vi "Open FTDI.vi"(8 "Baud Rate":u32=50000) -> (0 "FT_Status":u32(ring) items=["FT_OK", "FT_INVALID_HANDLE", "FT_DEVICE_NOT_FOUND", "FT_DEVICE_NOT_OPENED", "FT_IO_ERROR", "FT_INSUFFICIENT_RESOURCES", "FT_INVALID_PARAMETER", "FT_INVALID_BAUD_RATE", "FT_DEVICE_NOT_OPENED_FOR_ERASE", "FT_DEVICE_NOT_OPENED_FOR_WRITE", "FT_FAILED_TO_WRITE_DEVICE", "FT_EEPROM_READ_FAILED", "FT_EEPROM_WRITE_FAILED", "FT_EEPROM_ERASE_FAILED", "FT_EEPROM_NOT_PRESENT", "FT_EEPROM_NOT_PROGRAMMED", "FT_INVALID_ARGS", "FT_NOT_SUPPORTED", "FT_OTHER_ERROR"], 3 "FTDI Handle":u32)   [LabVIEW 2011, in "NMR.lvclass"]
uses:
  NMR.lvclass
panel:
  out "Device Description":string="FT232R USB UART"
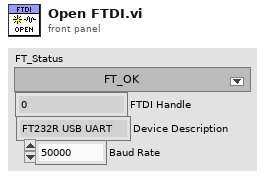
[diagram p1: front panel]
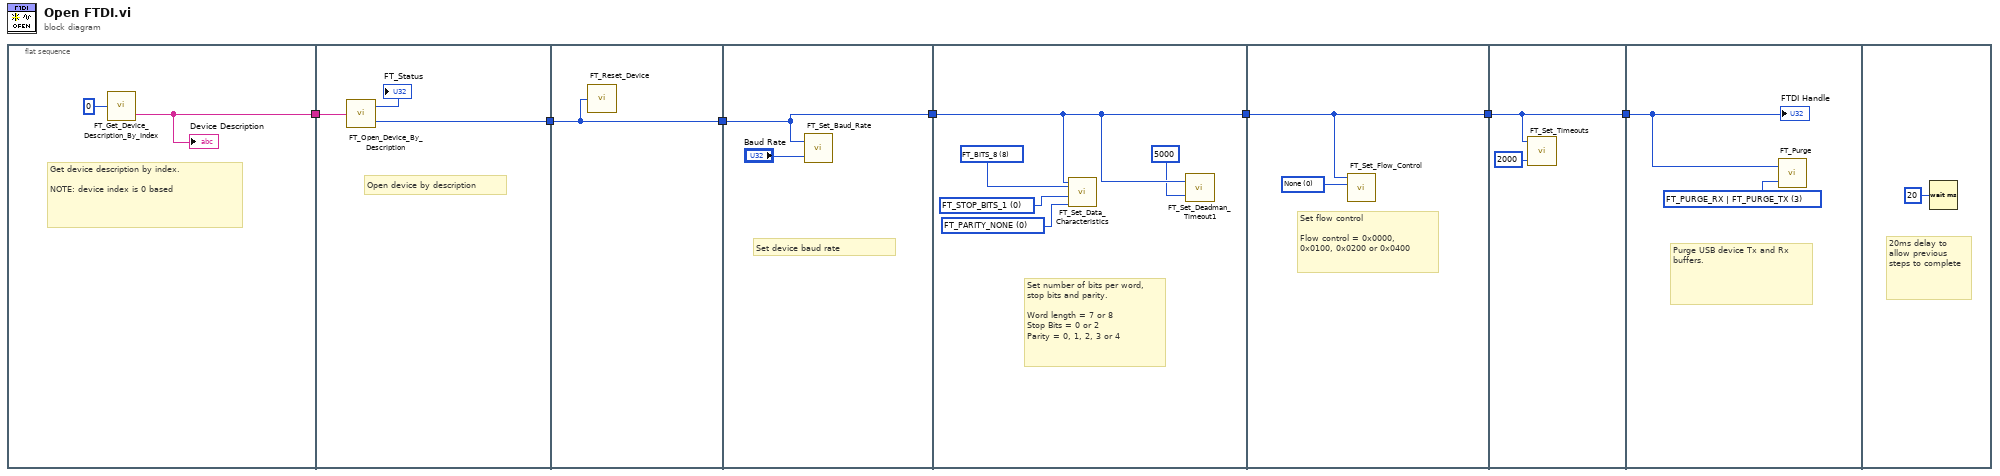
[diagram p0: block diagram]
diagram:
  n1 = flat-sequence {
    tunnel: [w8] -> w7
    tunnel: [w12] -> w6
    tunnel: w7 -> [w11]
    tunnel: w6 -> [w13]
    tunnel: [w13] -> w5
    tunnel: w5 -> [w14]
    tunnel: [w14] -> w4
    tunnel: w4 -> [w17]
    tunnel: [w17] -> w3
    tunnel: w3 -> [w22]
    tunnel: [w22] -> w2
    tunnel: w2 -> [w24]
    tunnel: [w24] -> w1
    tunnel: w1 -> [w26]
    frame #0 {
      # "Get device description by index.\n\nNOTE: device index is 0 based"
      n2 = call <instrlib>:"FT_Get_Device_Description_By_Index.vi"("Device Index"=u32 0) -> ("Device Description"=w8:string)  [unwired: 1 out]
      "Device Description" <- w8
    }
    frame #1 {
      # "Open device by description"
      n3 = call <instrlib>:"FT_Open_Device_By_Description.vi"("Device Description"=w11) -> ("FT_Status"=→"FT_Status":u32, "Handle"=w12:u32)
    }
    frame #2 {
      n4 = call <instrlib>:"FT_Reset_Device.vi"("Handle"=w13) -> ()  [unwired: 1 out]
    }
    frame #3 {
      # "Set device baud rate"
      n5 = call <instrlib>:"FT_Set_Baud_Rate.vi"("Baud Rate"="Baud Rate", "Handle"=w14) -> ()  [unwired: 1 out]
    }
    frame #4 {
      w19 = u8 0 items=["FT_PARITY_NONE", "FT_PARITY_ODD", "FT_PARITY_EVEN", "FT_PARITY_MARK", "FT_PARITY_SPACE"] ("Parity")
      w20 = u8 0 items=["FT_STOP_BITS_1"=0, "FT_STOP_BITS_2"=2] ("Stop Bits")
      w18 = u8 8 items=["FT_BITS_7"=7, "FT_BITS_8"=8] ("Word Length")
      # "Set number of bits per word, stop bits and parity.\n\nWord length = 7 or 8\nStop Bits = 0 or 2\nParity = 0, 1, 2, 3 or 4"
      n6 = call <instrlib>:"FT_Set_Data_Characteristics.vi"("Parity"=w19, "Stop Bits"=w20, "Word Length"=w18, "Handle"=w17) -> ()  [unwired: 1 out]
      n7 = call <instrlib>:"FT_Set_Deadman_Timeout1.vi"("DeadmanTimeout"=u32 5000, "Handle"=w17) -> ()  [unwired: 1 out]
    }
    frame #5 {
      w21 = u16 0 items=["None"=0, "RTS-CTS"=256, "DTR-DSR"=512, "XOn-XOff"=1024] ("Flow Control")
      # "Set flow control\n\nFlow control = 0x0000, 0x0100, 0x0200 or 0x0400"
      n8 = call <instrlib>:"FT_Set_Flow_Control.vi"("Flow Control"=w21, "Handle"=w22) -> ()  [unwired: 2 in, 1 out]
    }
    frame #6 {
      n9 = call <instrlib>:"FT_Set_Timeouts.vi"("Write Timeout"=u32 2000, "Handle"=w24) -> ()  [unwired: 1 in, 1 out]
    }
    frame #7 {
      w25 = u32 3 items=["FT_PURGE_RX"=1, "FT_PURGE_TX"=2, "FT_PURGE_RX | FT_PURGE_TX"=3] ("Purge Flags")
      # "Purge USB device Tx and Rx  buffers."
      n10 = call <instrlib>:"FT_Purge.vi"("Purge Flags"=w25, "Handle"=w26) -> ()  [unwired: 1 out]
      "FTDI Handle" <- w26
    }
    frame #8 {
      # "20ms delay to allow previous steps to complete"
      n11 = Wait (ms)(milliseconds to wait=u32 20) -> ()  [unwired: 1 out]
    }
  }
